vi "Process_Web_Services.vi"(8 "error in (no error)":errorcluster, 11 "IB_MSI in":refnum<class "IB_MSI.lvclass">) -> (0 "error out":errorcluster, 3 "IB_MSI out":refnum<class "IB_MSI.lvclass">)   [LabVIEW 2020, in "IB_MSI.lvclass"]
uses:
  <vilib>/AppBuilder/IB_Classes/MSI/IB_MSI.lvclass
  <vilib>/AppBuilder/IB_Classes/MSI/IB_MSI.lvclass/IB_MSI.ctl
  <vilib>/AppBuilder/IB_Classes/Installer/Installer.lvclass
  <vilib>/AppBuilder/IB_Classes/Source/IB_Source.lvclass
  <vilib>/AppBuilder/IB_Classes/Post_Install_Step/IB_Post_Install_Step.lvclass
  e:/builds/penguin/labview/branches/2020/dev/dist/vi.lib/AppBuilder/IB_Classes/Installer/Installer.lvclass
  e:/builds/penguin/labview/branches/2020/dev/dist/vi.lib/AppBuilder/IB_Classes/MSI/IB_MSI.lvclass
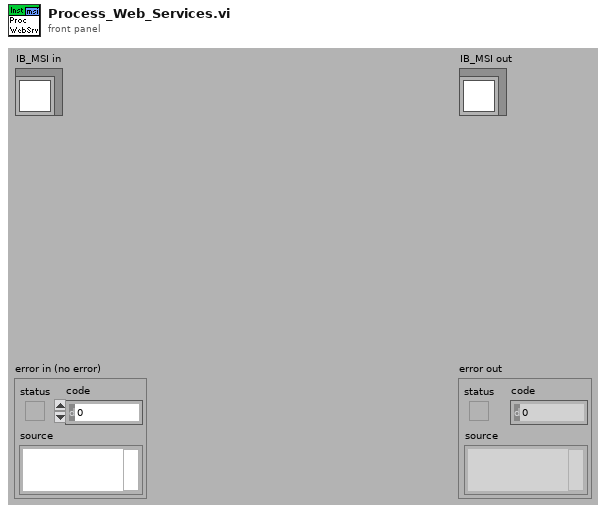
[diagram p1: front panel]
types:
  T1 = typedef "IB_Installer.ctl" = cluster{"Destination":refnum<class "IB_Destination.lvclass">[], "Source":refnum<class "IB_Source.lvclass">[], "buildObject":T2, "defaultDir":string, "platform":string, "author":string, "productName":string, "buildSpecName":string, "hide":bool, "requireLVDevSys":bool, "autoIncrement":bool, "includeError":bool, "readmeID":string, "buildLocation":path, "readmePath":path, "mediaSize":u16, "language":T3, "productVersion":T4, "preview":bool, "programmatic":bool, "progressBarEvents":T5, "userLog_Path":path, "shortcutAddresses":T7[], "EXE_Install Address":string, "EXE_Uninstall Address":string, "additional NIPaths":refnum<class "Dest_NI_NIPath.lvclass">[], "web service itemIDs":string[], "installerName":string}
  T2 = typedef "ItemRef.ctl" = u64
  T3 = typedef "CDK_sTypeDef_Languages.ctl" = u16
  T4 = typedef "CDK_sTypeDef_ProductVersion.ctl" = cluster{"Major":u8, "Minor":u8, "Update":u16}
  T5 = typedef "provcom_ProgressBar_Events.ctl" = cluster{"newJob":refnum<user-event>, "newItem":refnum<user-event>, "errorMsg":T6, "cancel":refnum<user-event>}
  T6 = typedef "mxLvBuildError.ctl" = refnum<user-event>
  T7 = typedef "CDK_sTypeDef_ShortcutAddress.ctl" = cluster{"file":string, "shortcut":string}
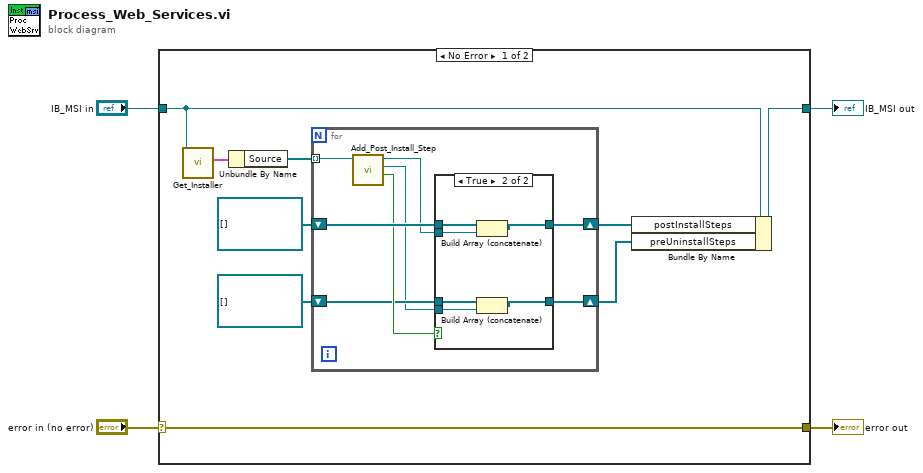
[diagram p0: block diagram]
diagram:
  n1 = case shown="No Error" "error in (no error)" {
    selector: "error in (no error)" -> [w13 w31]
    tunnel: [w13 w31] -> w1
    tunnel: [w10 w30] -> w3
    tunnel: "IB_MSI in" -> [w9 w30]
    frame No Error {
      n2 = call <vilib>:"Get_Installer.vi"("Installer in"=w9) -> ("data"=w8:T1)  [unwired: 1 in, 9 out]
      n3 = Unbundle By Name(w8) -> ("Source"=w12:refnum<class "IB_Source.lvclass">[])
      n4 = for {
        tunnel: w12 -> [w21] mode=indexing
        shift-right: [w19] -> w11
        shift-left: refnum<class "IB_Post_Install_Step.lvclass">[] [] -> [w20]
        shift-right: [w15] -> w5
        shift-left: refnum<class "IB_Post_Install_Step.lvclass">[] [] -> [w16]
        n5 = call-dynamic "Add_Post_Install_Step.vi"("IB_Source in"=w21) -> ("add?"=w17:bool, "Pre_Uninstall_Step"=w14:refnum<class "IB_Post_Install_Step.lvclass">, "Post_Install_Step"=w18:refnum<class "IB_Post_Install_Step.lvclass">)  [unwired: 1 in, 7 out]
        n6 = case shown="True" w17 {
          tunnel: w20 -> [w23 w29]
          tunnel: [w23 w28] -> w19
          tunnel: w18 -> [_ w27]
          tunnel: w16 -> [w22 w26]
          tunnel: [w22 w25] -> w15
          tunnel: w14 -> [_ w24]
          frame False {
          }
          frame True {
            n7 = Build Array (concatenate)(w29, w27) -> (w28:refnum<class "IB_Post_Install_Step.lvclass">[])
            n8 = Build Array (concatenate)(w26, w24) -> (w25:refnum<class "IB_Post_Install_Step.lvclass">[])
          }
        }
      }
      n9 = Bundle By Name(cluster=w9, "postInstallSteps"=w11, "preUninstallSteps"=w5) -> (w10:refnum<class "IB_MSI.lvclass">)
    }
    frame Error {
    }
  }
  "error out" <- w1
  "IB_MSI out" <- w3
